vi "Motor Control Global.vi"() -> ()   [LabVIEW 2009]
uses:
  Strict Lidar Motor Control Cluster.ctl
  Strict Raw Encoder Cluster.ctl
  Strict Drive Motor Control Cluster.ctl
  Strict Steering Motor Control Cluster.ctl
  Strict Lidar Motor Indicator Cluster.ctl
  Strict Steering Motor Indicator Cluster.ctl
  Strict Custom Compensator.ctl
panel:
  in  "Lidar Encoder Zeroed from the Real Index":i32
  out "Mult 3: Writing Index":u32
  out "Mult 2: Writing Index":u32
  out "Mult 1: Writing Index":u32
  in  "Custom Compensator":T1={"Zero coefficients"=[0.0, 0.0, 0.0, 0.0, 0.0, 0.0], "Pole coefficients"=[0.0, 0.0, 0.0, 0.0, 0.0, 0.0], "Gain"=0.0}
  out "Drive Motor Indicator":T2
  out "Steering Motor Indicator":T3
  out "Lidar Motor Indicator":T4
  in  "Steering Motor Control":T5 {"Motor Voltage" format="%.17g"}
  in  "Drive Motor Control":T6 {"Motor Voltage" format="%.17g"}
  out "Encoder Information":T7
  in  "Lidar Motor Control":T8={"Reset Encoder"=FALSE, "Motor Enable"=FALSE, "Choice of Control Type"=enum."Direct Voltage Control", "Choice of Oscillation"=enum."Oscillate Voltage", "Choice of Compensation"=enum."None", "Choice of Error"=enum."Gray Error", "Units of pi rad 18b (s-fxp-1)"={"Phi_B Set Point (pi rad)"=0.0, "Phi_A Set Point (pi rad)"=0.0, "Phi_Lidar Set Point (pi rad)"=0.0, "Phi_Lidar - Phi_A"=0.0, "Phi_mass-Phi_Lidar"=0.0, "Convert (enc) to (pi rad)"=0.0, "Oscillation Frequency (pi rad per 100KHz)"=0.0}, "Units of 18b (s-fxp-1) gain"={"Proportional Gain"=0.0, " Integral Gain"=0.0, "Oscillation Setpoint Amplitude"=0.0, "Gravity Compensation Gain"=0.0, "Phi_B Set Point (enc) pre-gain"=0.0, "Phi_B Set Point (pi rad) pre-gain"=0.0, "Phi_A Set Point (pi rad) pre-gain"=0.0, "Phi_Lidar Set Point (pi rad) pre-gain"=0.0, "Derivative Gain"=0.0, "Double Integral Gain"=0.0, "Second Derivative Gain"=0.0}, "Units of 20b s-fxp-5 Voltage"={"Oscillation Voltage Amplitude"=0.0, "Motor Voltage"=0.0}, "Units of encoder 32b uint"={"Phi_B Set Point (enc)"=0, "Lidar Encoder Cap"=0}, "Debug Args"=[FALSE, FALSE, FALSE, FALSE, FALSE, FALSE, FALSE, FALSE, FALSE, FALSE, FALSE, FALSE, FALSE, FALSE, FALSE, FALSE, FALSE, FALSE, FALSE, FALSE], "Units of 8b int gain exponents"={"Proportional Gain"=0, " Integral Gain"=0, "Oscillation Setpoint Amplitude"=0, "Gravity Compensation Gain"=0, "Phi_B Set Point (enc) pre-gain"=0, "Phi_B Set Point (pi rad) pre-gain"=0, "Phi_A Set Point (pi rad) pre-gain"=0, "Phi_Lidar Set Point (pi rad) pre-gain"=0, "Derivative Gain"=0, "Double Integral Gain"=0, "Second Derivative Gain"=0}, "6b (u-fxp-6)"={"Size of Integrator"=0.0, "Size of IIntigrator"=0.0, "Size of Differentiator"=0.0, "Size of DDifferentiator"=0.0}} {"Units of 20b s-fxp-5 Voltage"."Motor Voltage" format="%.17g"}
  in  "Drive Speed, Measured (ft/sec)":fxp<+/-,14,4>
  in  "stop":bool
  in  "Lidar Encoder":i32
  in  "Steering Encoder":i32
  in  "Drive Encoder":i32
  # "Phi_B is the Motor Crank\nPhi_A is the Rocker\n\nBoth are in units of pi radians \nand both are encoded in format\n18b s-fxp-1"
  # "X must be zero for this code to work.\nOtherwise I would have to redo the\nlookup tables for the new X"
  # "50 Hz Update Frequency"
  # "50 Hz Update Frequency"
  # "50Hz Update Frequency"
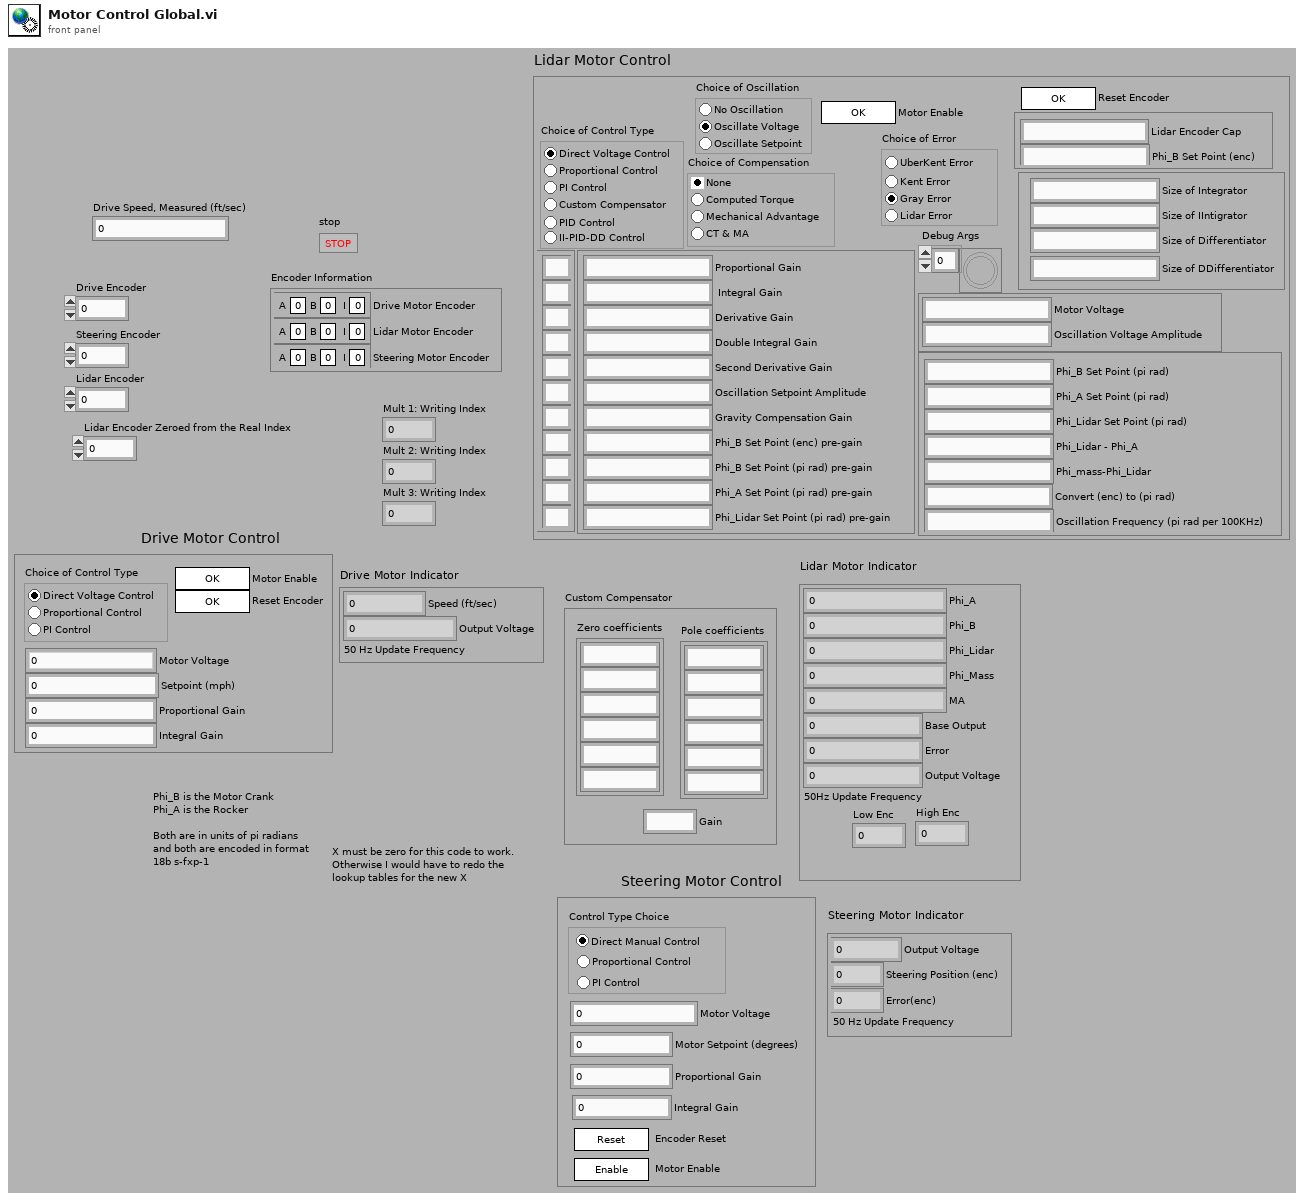
[diagram p1: front panel]
types:
  T1 = typedef "Strict Custom Compensator.ctl" = cluster{"Zero coefficients":fxp<+/-,18,1>[], "Pole coefficients":fxp<+/-,18,1>[], "Gain":fxp<+/-,18,1>}
  T2 = cluster{"Speed (ft/sec)":fxp<+/-,14,4>, "Output Voltage":fxp<+/-,20,5>}
  T3 = typedef "Strict Steering Motor Indicator Cluster.ctl" = cluster{"Output Voltage":fxp<+/-,20,5>, "Steering Position (enc)":i32, "Error(enc)":i32}
  T4 = typedef "Strict Lidar Motor Indicator Cluster.ctl" = cluster{"Phi_A":fxp<+/-,18,1>, "Phi_B":fxp<+/-,18,1>, "Output Voltage":fxp<+/-,20,5>, "Phi_Lidar":fxp<+/-,18,1>, "Phi_Mass":fxp<+/-,18,1>, "MA":fxp<+/-,18,1>, "Base Output":fxp<+/-,18,1>, "Error":fxp<+/-,18,1>, "Low Enc":i32, "High Enc":i32}
  T5 = typedef "Strict Steering Motor Control Cluster.ctl" = cluster{"Encoder Reset":bool, "Motor Voltage":fxp<+/-,20,5>, "Proportional Gain":fxp<+/-,20,5>, "Motor Setpoint (degrees)":i32, "Control Type Choice":enum32{"Direct Manual Control", "Proportional Control", "PI Control"}, "Integral Gain":fxp<+/-,20,5>, "Motor Enable":bool}
  T6 = typedef "Strict Drive Motor Control Cluster.ctl" = cluster{"Motor Voltage":fxp<+/-,20,5>, "Setpoint (mph)":fxp<+/-,20,7>, "Proportional Gain":fxp<+/-,20,5>, "Choice of Control Type":enum32{"Direct Voltage Control", "Proportional Control", "PI Control"}, "Integral Gain":fxp<+/-,20,5>, "Reset Encoder":bool, "Motor Enable":bool}
  T7 = typedef "Strict Raw Encoder Cluster.ctl" = cluster{"Drive Motor Encoder":cluster{"A":bool, "B":bool, "I":bool}, "Lidar Motor Encoder":cluster{"A":bool, "B":bool, "I":bool}, "Steering Motor Encoder":cluster{"A":bool, "B":bool, "I":bool}}
  T8 = typedef "Strict Lidar Motor Control Cluster.ctl" = cluster{"Reset Encoder":bool, "Motor Enable":bool, "Choice of Control Type":enum32{"Direct Voltage Control", "Proportional Control", "PI Control", "Custom Compensator", "PID Control", "II-PID-DD Control"}, "Choice of Oscillation":enum32{"Oscillate Voltage", "Oscillate Setpoint", "No Oscillation"}, "Choice of Compensation":enum32{"None", "Computed Torque", "Mechanical Advantage", "CT & MA "}, "Choice of Error":enum32{"Gray Error", "Lidar Error", "Kent Error", "UberKent Error"}, "Units of pi rad 18b (s-fxp-1)":cluster{"Phi_B Set Point (pi rad)":fxp<+/-,18,1>, "Phi_A Set Point (pi rad)":fxp<+/-,18,1>, "Phi_Lidar Set Point (pi rad)":fxp<+/-,18,1>, "Phi_Lidar - Phi_A":fxp<+/-,18,1>, "Phi_mass-Phi_Lidar":fxp<+/-,18,1>, "Convert (enc) to (pi rad)":fxp<+/-,18,1>, "Oscillation Frequency (pi rad per 100KHz)":fxp<+/-,18,1>}, "Units of 18b (s-fxp-1) gain":cluster{"Proportional Gain":fxp<+/-,18,1>, " Integral Gain":fxp<+/-,18,1>, "Oscillation Setpoint Amplitude":fxp<+/-,18,1>, "Gravity Compensation Gain":fxp<+/-,18,1>, "Phi_B Set Point (enc) pre-gain":fxp<+/-,18,1>, "Phi_B Set Point (pi rad) pre-gain":fxp<+/-,18,1>, "Phi_A Set Point (pi rad) pre-gain":fxp<+/-,18,1>, "Phi_Lidar Set Point (pi rad) pre-gain":fxp<+/-,18,1>, "Derivative Gain":fxp<+/-,18,1>, "Double Integral Gain":fxp<+/-,18,1>, "Second Derivative Gain":fxp<+/-,18,1>}, "Units of 20b s-fxp-5 Voltage":cluster{"Oscillation Voltage Amplitude":fxp<+/-,20,5>, "Motor Voltage":fxp<+/-,20,5>}, "Units of encoder 32b uint":cluster{"Phi_B Set Point (enc)":i32, "Lidar Encoder Cap":i32}, "Debug Args":bool[], "Units of 8b int gain exponents":cluster{"Proportional Gain":i8, " Integral Gain":i8, "Oscillation Setpoint Amplitude":i8, "Gravity Compensation Gain":i8, "Phi_B Set Point (enc) pre-gain":i8, "Phi_B Set Point (pi rad) pre-gain":i8, "Phi_A Set Point (pi rad) pre-gain":i8, "Phi_Lidar Set Point (pi rad) pre-gain":i8, "Derivative Gain":i8, "Double Integral Gain":i8, "Second Derivative Gain":i8}, "6b (u-fxp-6)":cluster{"Size of Integrator":fxp<+,6,6>, "Size of IIntigrator":fxp<+,6,6>, "Size of Differentiator":fxp<+,6,6>, "Size of DDifferentiator":fxp<+,6,6>}}
diagram:
